vi "(SubVI)Control Data_Save or Load Caller's Control Value.vi"(6 "Common?":bool, 7 "Function":T1, 8 "error in (no error)":errorcluster caption="에러 입력(에러 없음)") -> (0 "error out":errorcluster caption="에러 출력")   [LabVIEW 2020]
uses:
  Controls/(Ctrl)Control Data_Save or Load Control Data_Function.ctl
  Variables/(Var)System Variables.vi
  <vilib>/Utility/config.llb/Write Key (String).vi
  <vilib>/Utility/config.llb/Read Key (String).vi
  <vilib>/Utility/config.llb/NI_LVConfig.lvlib
panel:
  # "(SubVI)Save or Load Caller's Control Value.vi By hspark\n\nDescription : 호출한 VI의 모든 컨트롤의 현재 값을 저장하거나, 저장된 값을 불러오는 VI\n\nInput : \n1. Function : 저장 또는 불러오기 동작 입력\n2. Common? : false 입력 시 Default Path에 Chip Type을 추가한 경로 사용\n\nOutput : \n\nLabVIEW Version : 2020 SP1 이상\n\nNote :\nINI 파일 형식을 사용함\n섹션 : 컨트롤/인디케이터의 소유자 VI\n키 : 컨트롤의 라벨\n값 : 배리언트 변환 후 패턴화\n\n* 컨트롤/인디케이터 라벨 또는 VI 이름 변경 시 저장된 값 불러오기 안됨\n\nUpdate : 2022.01.06"
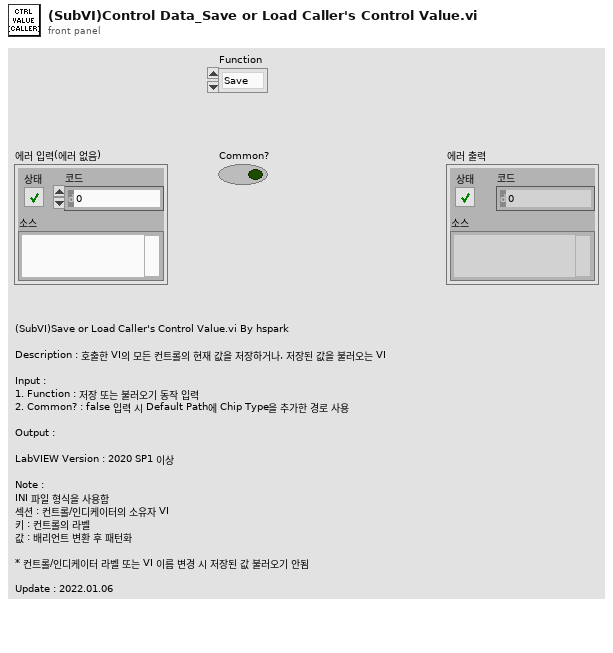
[diagram p1: front panel]
types:
  T1 = typedef "(Ctrl)Control Data_Save or Load Control Data_Function.ctl" = enum16{"Save", "Load"}
  T2 = typedef "Haptic IC.lvclass/(Ctrl)IC Type.ctl" = enum8{"DW7800", "DW7802", "DW7912", "DW7914"}
  T3 = typedef "NI_LVConfig.lvlib/Config Data RefNum.ctl" = refnum<k1>
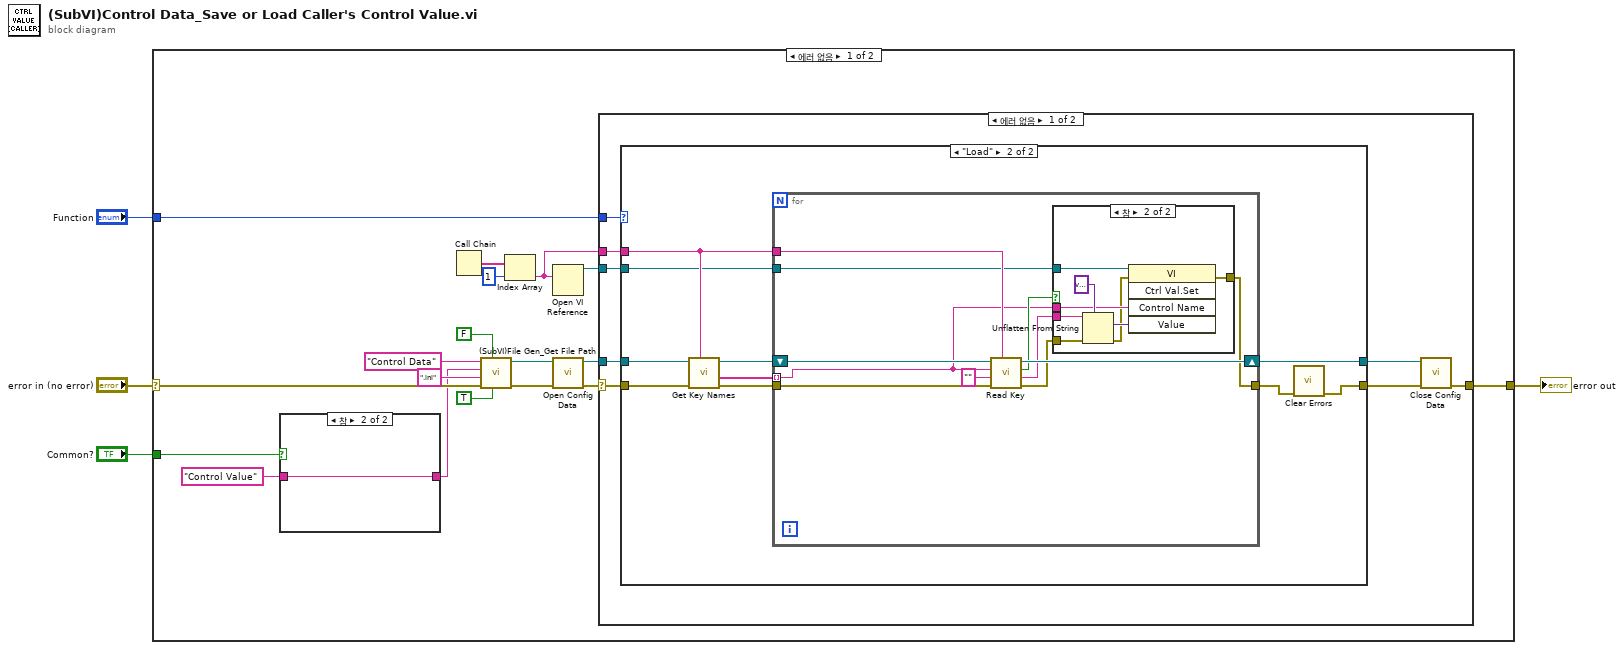
[diagram p0: block diagram]
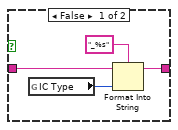
[diagram p2: hidden frame]
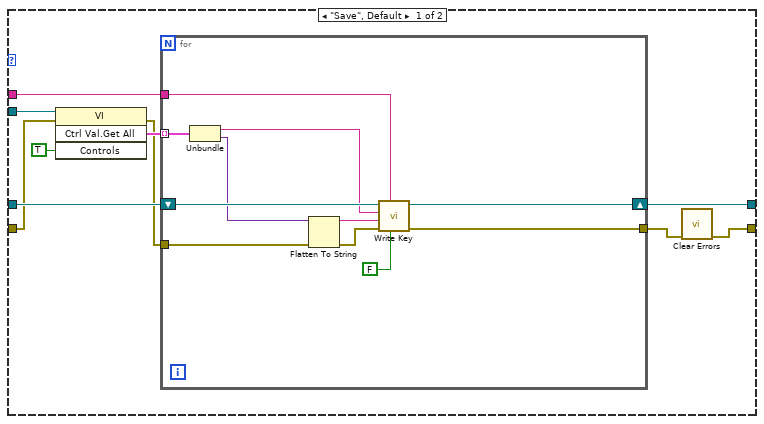
[diagram p3: hidden frame]
diagram:
  n1 = case shown="에러 없음" "error in (no error)" {
    selector: "error in (no error)" -> [w16 w88]
    tunnel: [w20 w88] -> w3
    tunnel: "Function" -> [w19 _]
    tunnel: "Common?" -> [w6 _]
    frame No Error {
      n2 = case shown="참" w6 {
        tunnel: "Control Value" -> [w25 w27]
        tunnel: [w23 w27] -> w7
        frame False {
          n3 = global read "(Var)System Variables.vi" "IC Type"() -> (w24:T2)
          n4 = Format Into String(format string="_%s" ("포맷 문자열"), initial string=w25, w24) -> (resulting string=w23:string)  [unwired: 1 in, 1 out]
        }
        frame True {
        }
      }
      n5 = Call Chain() -> (call chain=w12:string[])
      n6 = call "(SubVI)File Gen_Get File Path.vi"("Common?"=TRUE ("Common? (f)"), "Use Timestamp"=FALSE, "error in (no error)"=w16, "File Extension (.txt)"=".ini", "File Name"=w7, "Folder Name"="Control Data") -> ("error out"=w15:errorcluster, "Path"=w14:path)  [unwired: 3 in, 1 out]
      n7 = Index Array(array=w12, index=1 ("인덱스")) -> (element=w10:string)
      n8 = Open VI Reference(vi path=w10) -> (vi reference=w11:refnum<vi>)  [unwired: 5 in, 1 out]
      n9 = call <vilib>:"Open Config Data.vi"("error in (no error)"=w15, "configuration file path"=w14) -> ("error out"=w21:errorcluster, "refnum"=w22:T3)  [unwired: 7 in, 1 out]
      n10 = case shown="에러 없음" w21 {
        selector: w21 -> [w33 w87]
        tunnel: w19 -> [w35 _]
        tunnel: w22 -> [w34 _]
        tunnel: [w31 w87] -> w20
        tunnel: w11 -> [w29 _]
        tunnel: w10 -> [w28 _]
        frame No Error {
          n11 = case shown="\"Load\"" w35 {
            tunnel: w34 -> [w45 w66]
            tunnel: w33 -> [w37 w61]
            tunnel: [w42 w63] -> w32
            tunnel: [w44 w65] -> w30
            tunnel: w29 -> [w41 w57]
            tunnel: w28 -> [w38 w60]
            frame "Save", Default {
              n12 = invoke class="VI" method="Ctrl Val.Get All"(reference=w41, error in=w37, "Controls"=TRUE ("컨트롤")) -> (error out=w36:errorcluster, "Get All Control Values Variant"=w39:cluster{"Name":string, "Variant Data":variant}[])  [unwired: 1 in, 2 out]
              n13 = for {
                shift-right: [w53] -> w44
                shift-left: w45 -> [w56]
                tunnel: [w51] -> w43
                tunnel: w39 -> [w49] mode=indexing
                tunnel: w38 -> [w50]
                tunnel: w36 -> [w46]
                n14 = Unbundle(w49) -> ("Name"=w48:string, "Variant Data"=w47:variant)
                n15 = Flatten To String(anything=w47, error in (no error)=w46) -> (data string=w55:string, error out=w54:errorcluster)  [unwired: 2 in, 1 out]
                n16 = call-poly <vilib>:"Write Key.vi"("write raw string? (F)"=FALSE, "section"=w50, "error in (no error)"=w54, "value"=w55, "key"=w48, "refnum"=w56) -> ("error out"=w51:errorcluster, "refnum out"=w53:T3)  [unwired: 3 in, 1 out]
              }
              n17 = call <vilib>:"Clear Errors.vi"("error in (no error)"=w43) -> ("error out"=w42:errorcluster)  [unwired: 5 in, 1 out]
            }
            frame "Load" {
              n18 = call <vilib>:"Get Key Names.vi"("section"=w60, "error in (no error)"=w61, "refnum"=w66) -> ("error out"=w59:errorcluster, "key names"=w58:string[], "refnum out"=w62:T3)  [unwired: 5 in, 1 out]
              n19 = for {
                shift-right: [w76] -> w65
                shift-left: w62 -> [w77]
                tunnel: [w67] -> w64
                tunnel: w60 -> [w75]
                tunnel: w59 -> [w74]
                tunnel: w58 -> [w68] mode=indexing
                tunnel: w57 -> [w70]
                n20 = call-poly <vilib>:"Read Key.vi"("section"=w75, "error in (no error)"=w74, "default value"="", "key"=w68, "refnum"=w77) -> ("error out"=w69:errorcluster, "value"=w71:string, "found?"=w73:bool, "refnum out"=w76:T3)  [unwired: 3 in]
                n21 = case shown="참" w73 {
                  tunnel: w71 -> [_ w86]
                  tunnel: w70 -> [_ w84]
                  tunnel: w69 -> [w78 w81]
                  tunnel: w68 -> [_ w82]
                  tunnel: [w78 w79] -> w67
                  frame False {
                  }
                  frame True {
                    n22 = Unflatten From String(type=variant, binary string=w86, error in (no error)=w81) -> (value=w83:variant, error out=w80:errorcluster)  [unwired: 2 in, 1 out]
                    n23 = invoke class="VI" method="Ctrl Val.Set"(reference=w84, error in=w80, "Control Name"=w82, "Value"=w83) -> (error out=w79:errorcluster)  [unwired: 1 in, 4 out]
                  }
                }
              }
              n24 = call <vilib>:"Clear Errors.vi"("error in (no error)"=w64) -> ("error out"=w63:errorcluster)  [unwired: 5 in, 1 out]
            }
          }
          n25 = call <vilib>:"Close Config Data.vi"("error in (no error)"=w32, "refnum"=w30) -> ("error out"=w31:errorcluster)  [unwired: 8 in, 1 out]
        }
        frame Error {
        }
      }
    }
    frame Error {
    }
  }
  "error out" <- w3
